vi "USRP_singlecarrierTDMUSRP1_withoutemu.vi"() -> ()   [LabVIEW 2021]
uses:
  <vilib>/addons/Modulation/Analog/controls/Complex Data Waveform.ctl
  <vilib>/Analysis/coordinate.llb/Angle Units.ctl
  <vilib>/Analysis/coordinate.llb/Angle Range (Degree).ctl
  <vilib>/Analysis/coordinate.llb/Wrap Angle (scalar).vi
  system stop.vi
  <vilib>/measure/matone.llb/Extract Single Tone Information 1 Chan (CDB).vi
  <instrlib>/niUSRP/niUSRP Fetch Rx Data (CDB Cluster).vi
  <instrlib>/niUSRP/niUSRP Write Tx Data (CDB Cluster).vi
  <vilib>/addons/Modulation/niAMT.lvlib
  <vilib>/measure/NI_MAPro.lvlib
  <vilib>/Analysis/NI_AAL_Angle.lvlib
panel:
  in  "Tab Control":T1(tab)
  in  "IQ rate Tx":dbl=400000.0 format="%#_6p"
  in  "Tx Gain":dbl format="%#_6f"
  in  "Tx IP":refnum<k15>="192.168.10.2"
  out "coerced IQ rate Tx":dbl=100000.0 format="%#_6p"
  out "coerced carrier frequency Tx":dbl=100000.0 format="%#_6p"
  in  "Rx IP":refnum<k15>="192.168.10.2"
  in  "Rx gain":dbl format="%#_6f"
  in  "Frequency":dbl=10000.0 format="%#_13g"
  in  "Duration":dbl=0.01 format="%#_13g"
  out "coerced IQ rate Rx":dbl=100000.0 format="%#_6p"
  out "coerced carrier frequency Rx":dbl=100000.0 format="%#_6p"
  in  "number of samples":i64=4000
  in  "carrier frequency":dbl=2400000000.0 format="%#_6p"
  in  "Phase in deg":dbl
  out "Waveform Graph":dbl[](graph)
  out "Boolean":bool
  out "detected frequency":dbl format="%.2p"
  out "detected Amplitude in dBm":dbl format="%.2p"
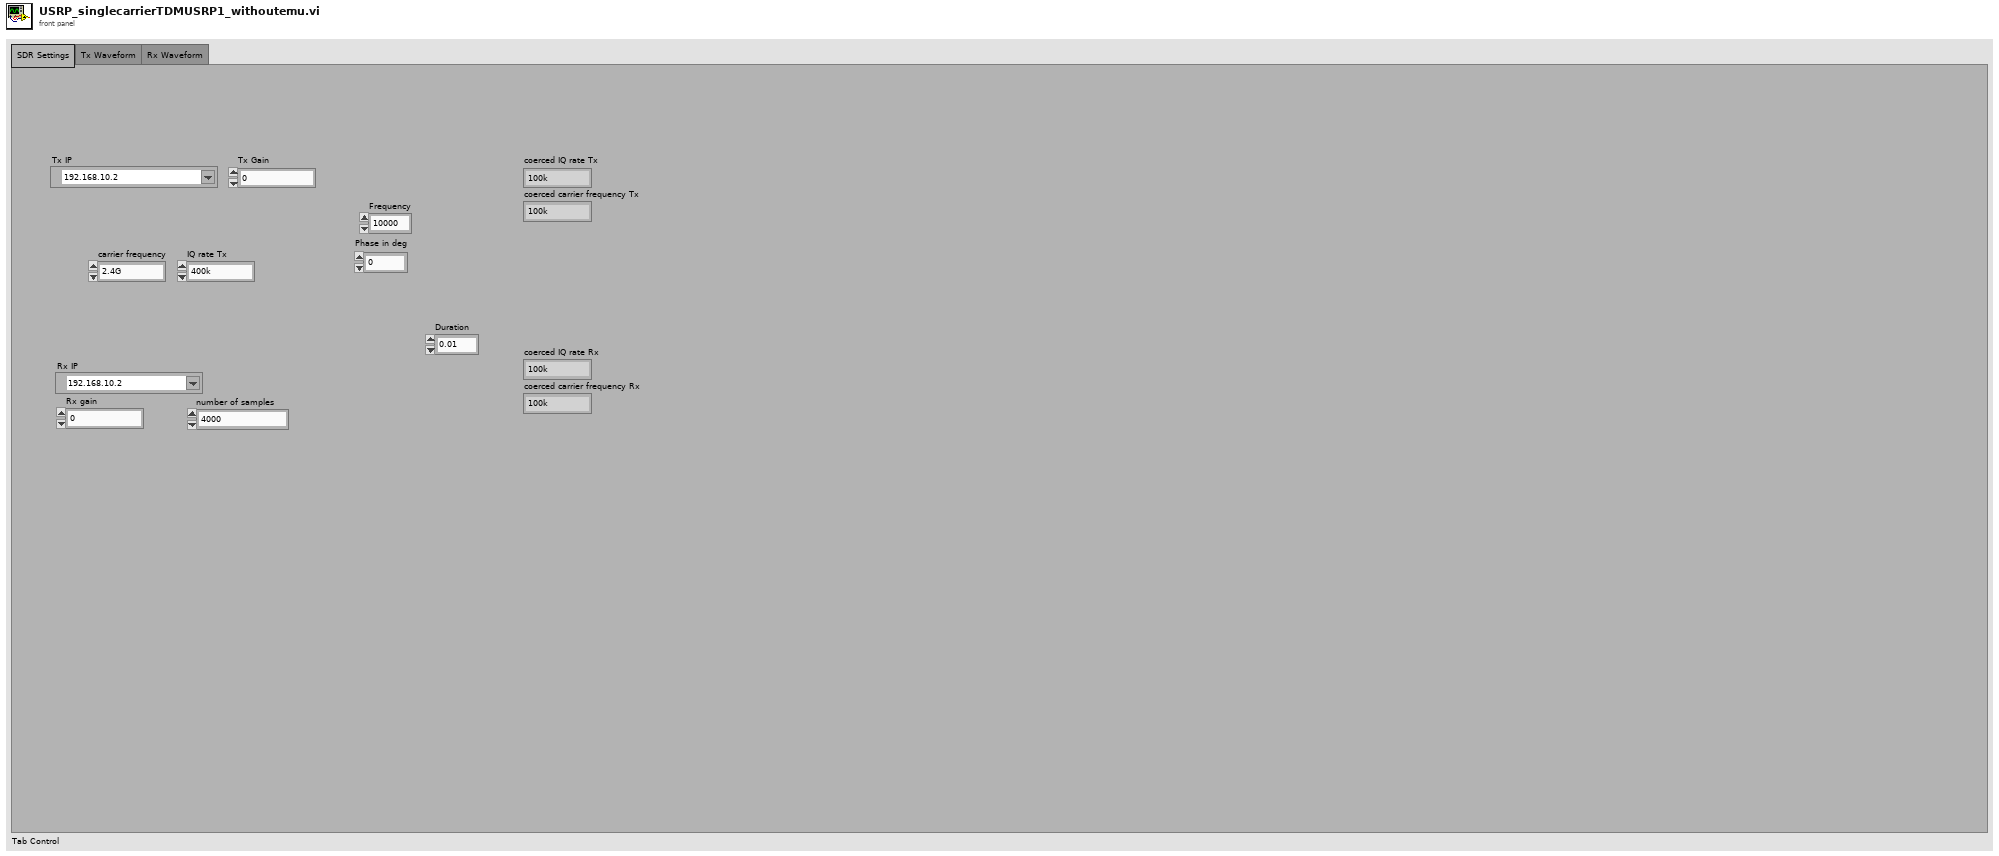
[diagram p1: front panel]
types:
  T1 = enum32{"SDR Settings", "Tx Waveform", "Rx Waveform"}
  T2 = typedef "niAMT.lvlib/Complex Data Waveform.ctl" = cluster{"t0":dbl, "dt":dbl, "Y":cdb[]}
  T3 = typedef "NI_AAL_Angle.lvlib/Angle Range (Degree).ctl" = u16
  T4 = typedef "NI_AAL_Angle.lvlib/Angle Units.ctl" = i32
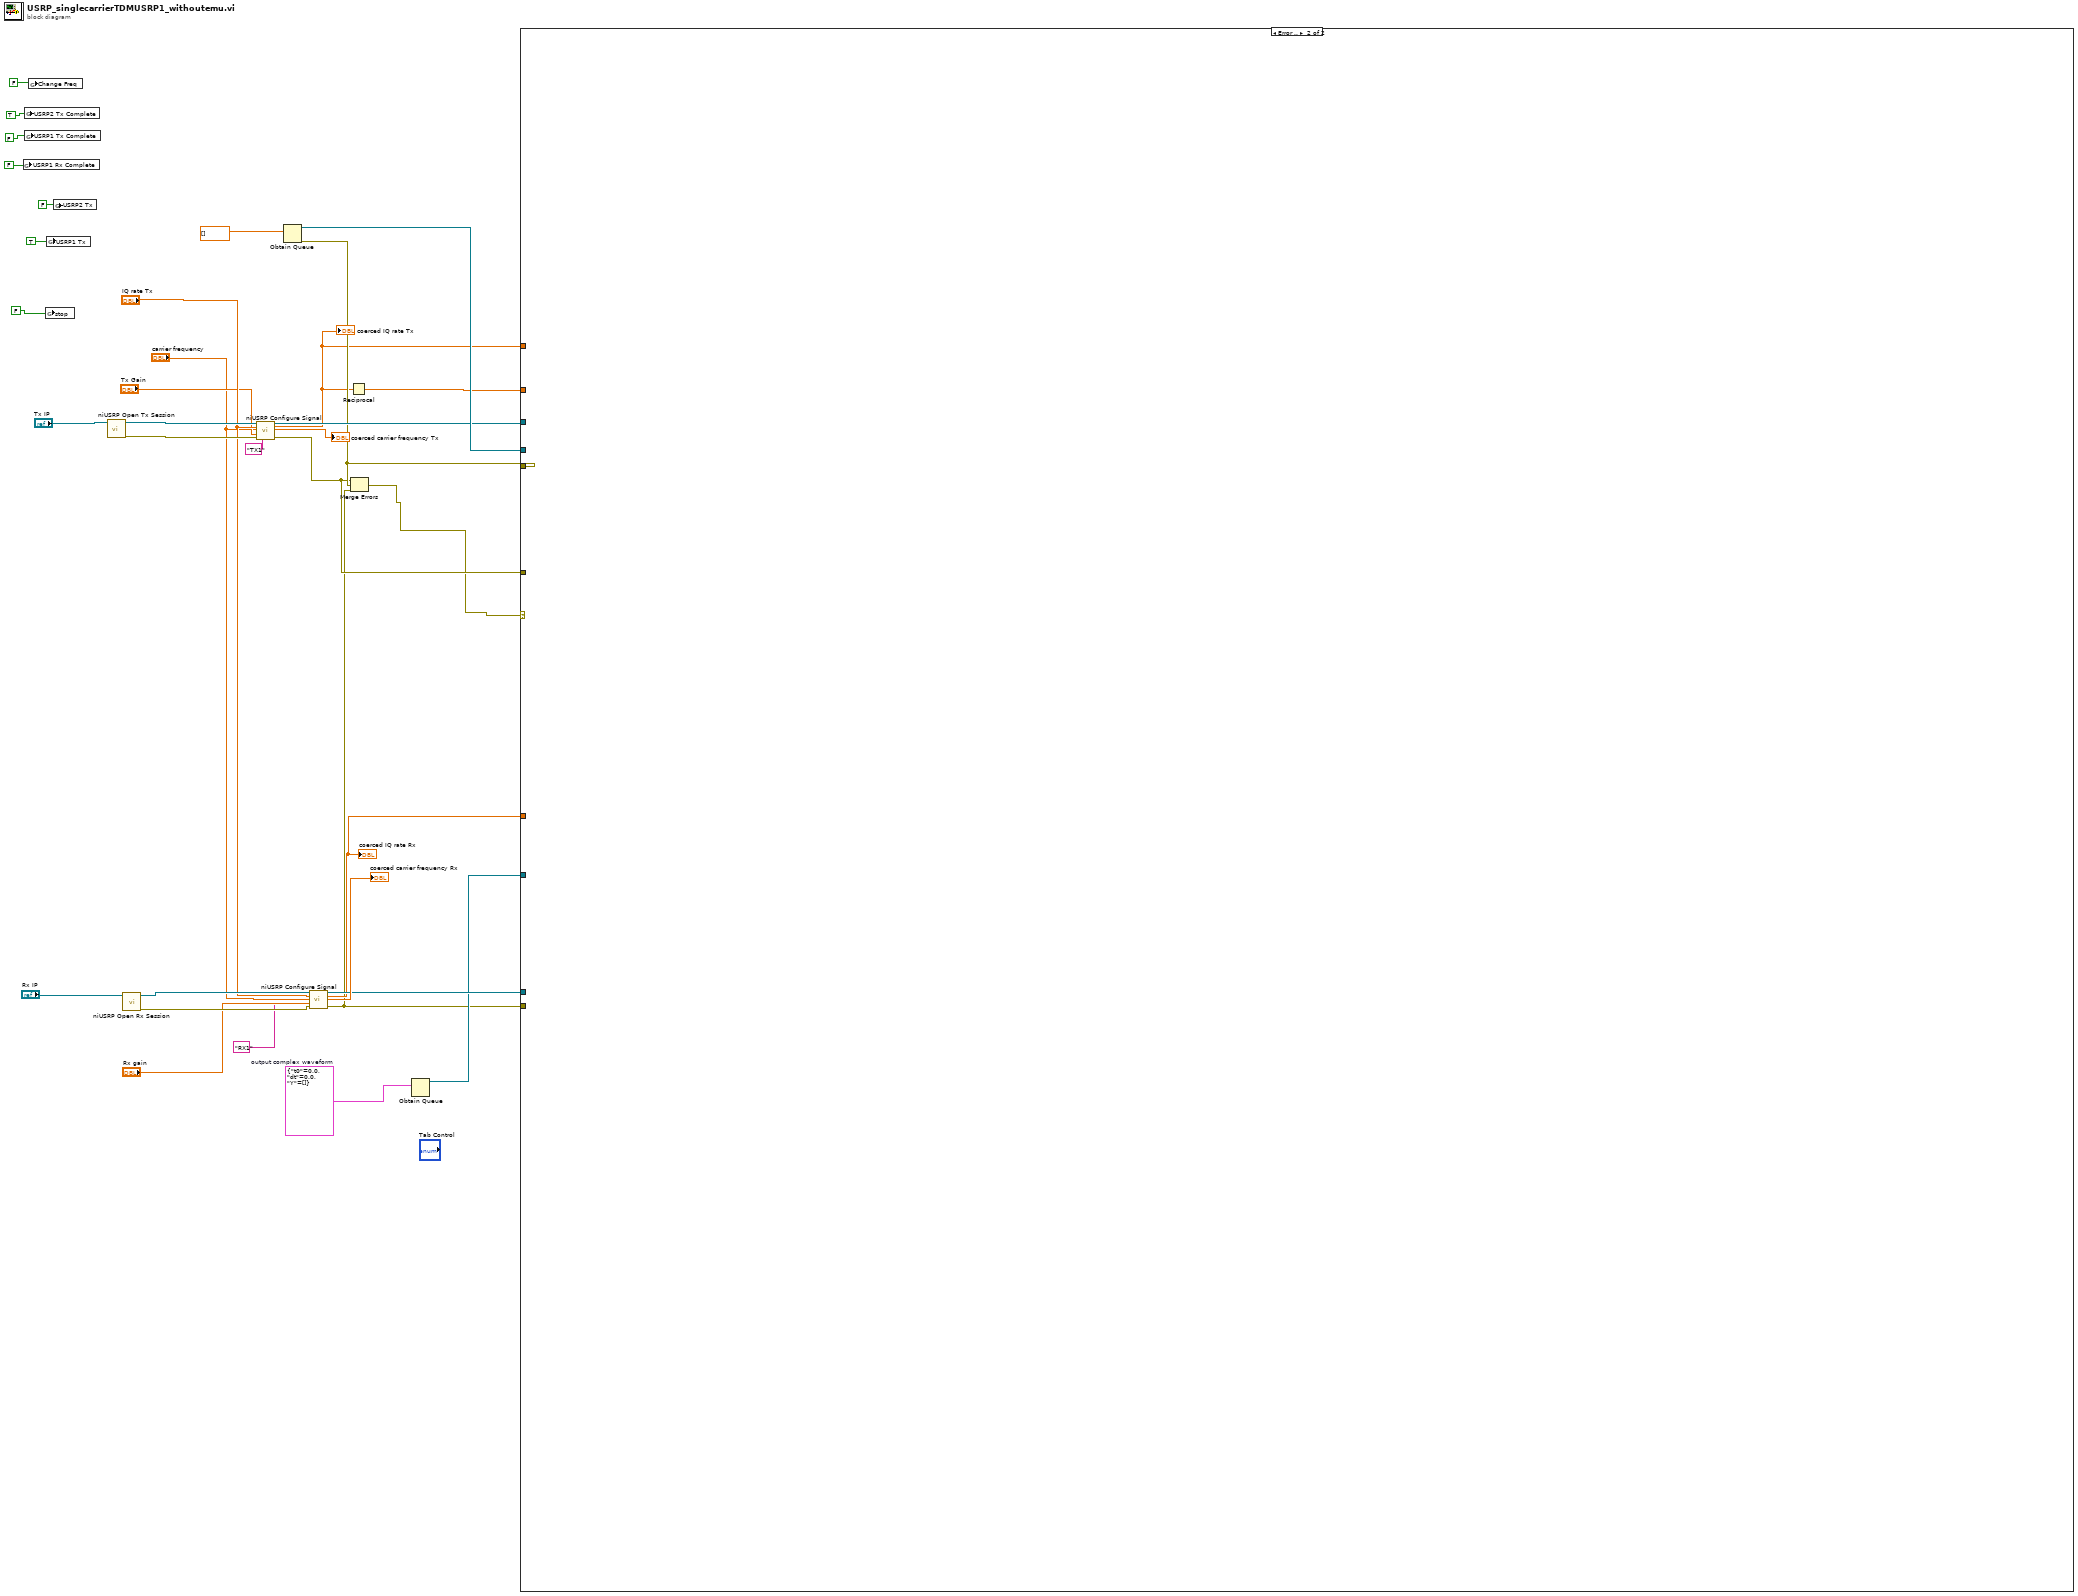
[diagram p0: block diagram]
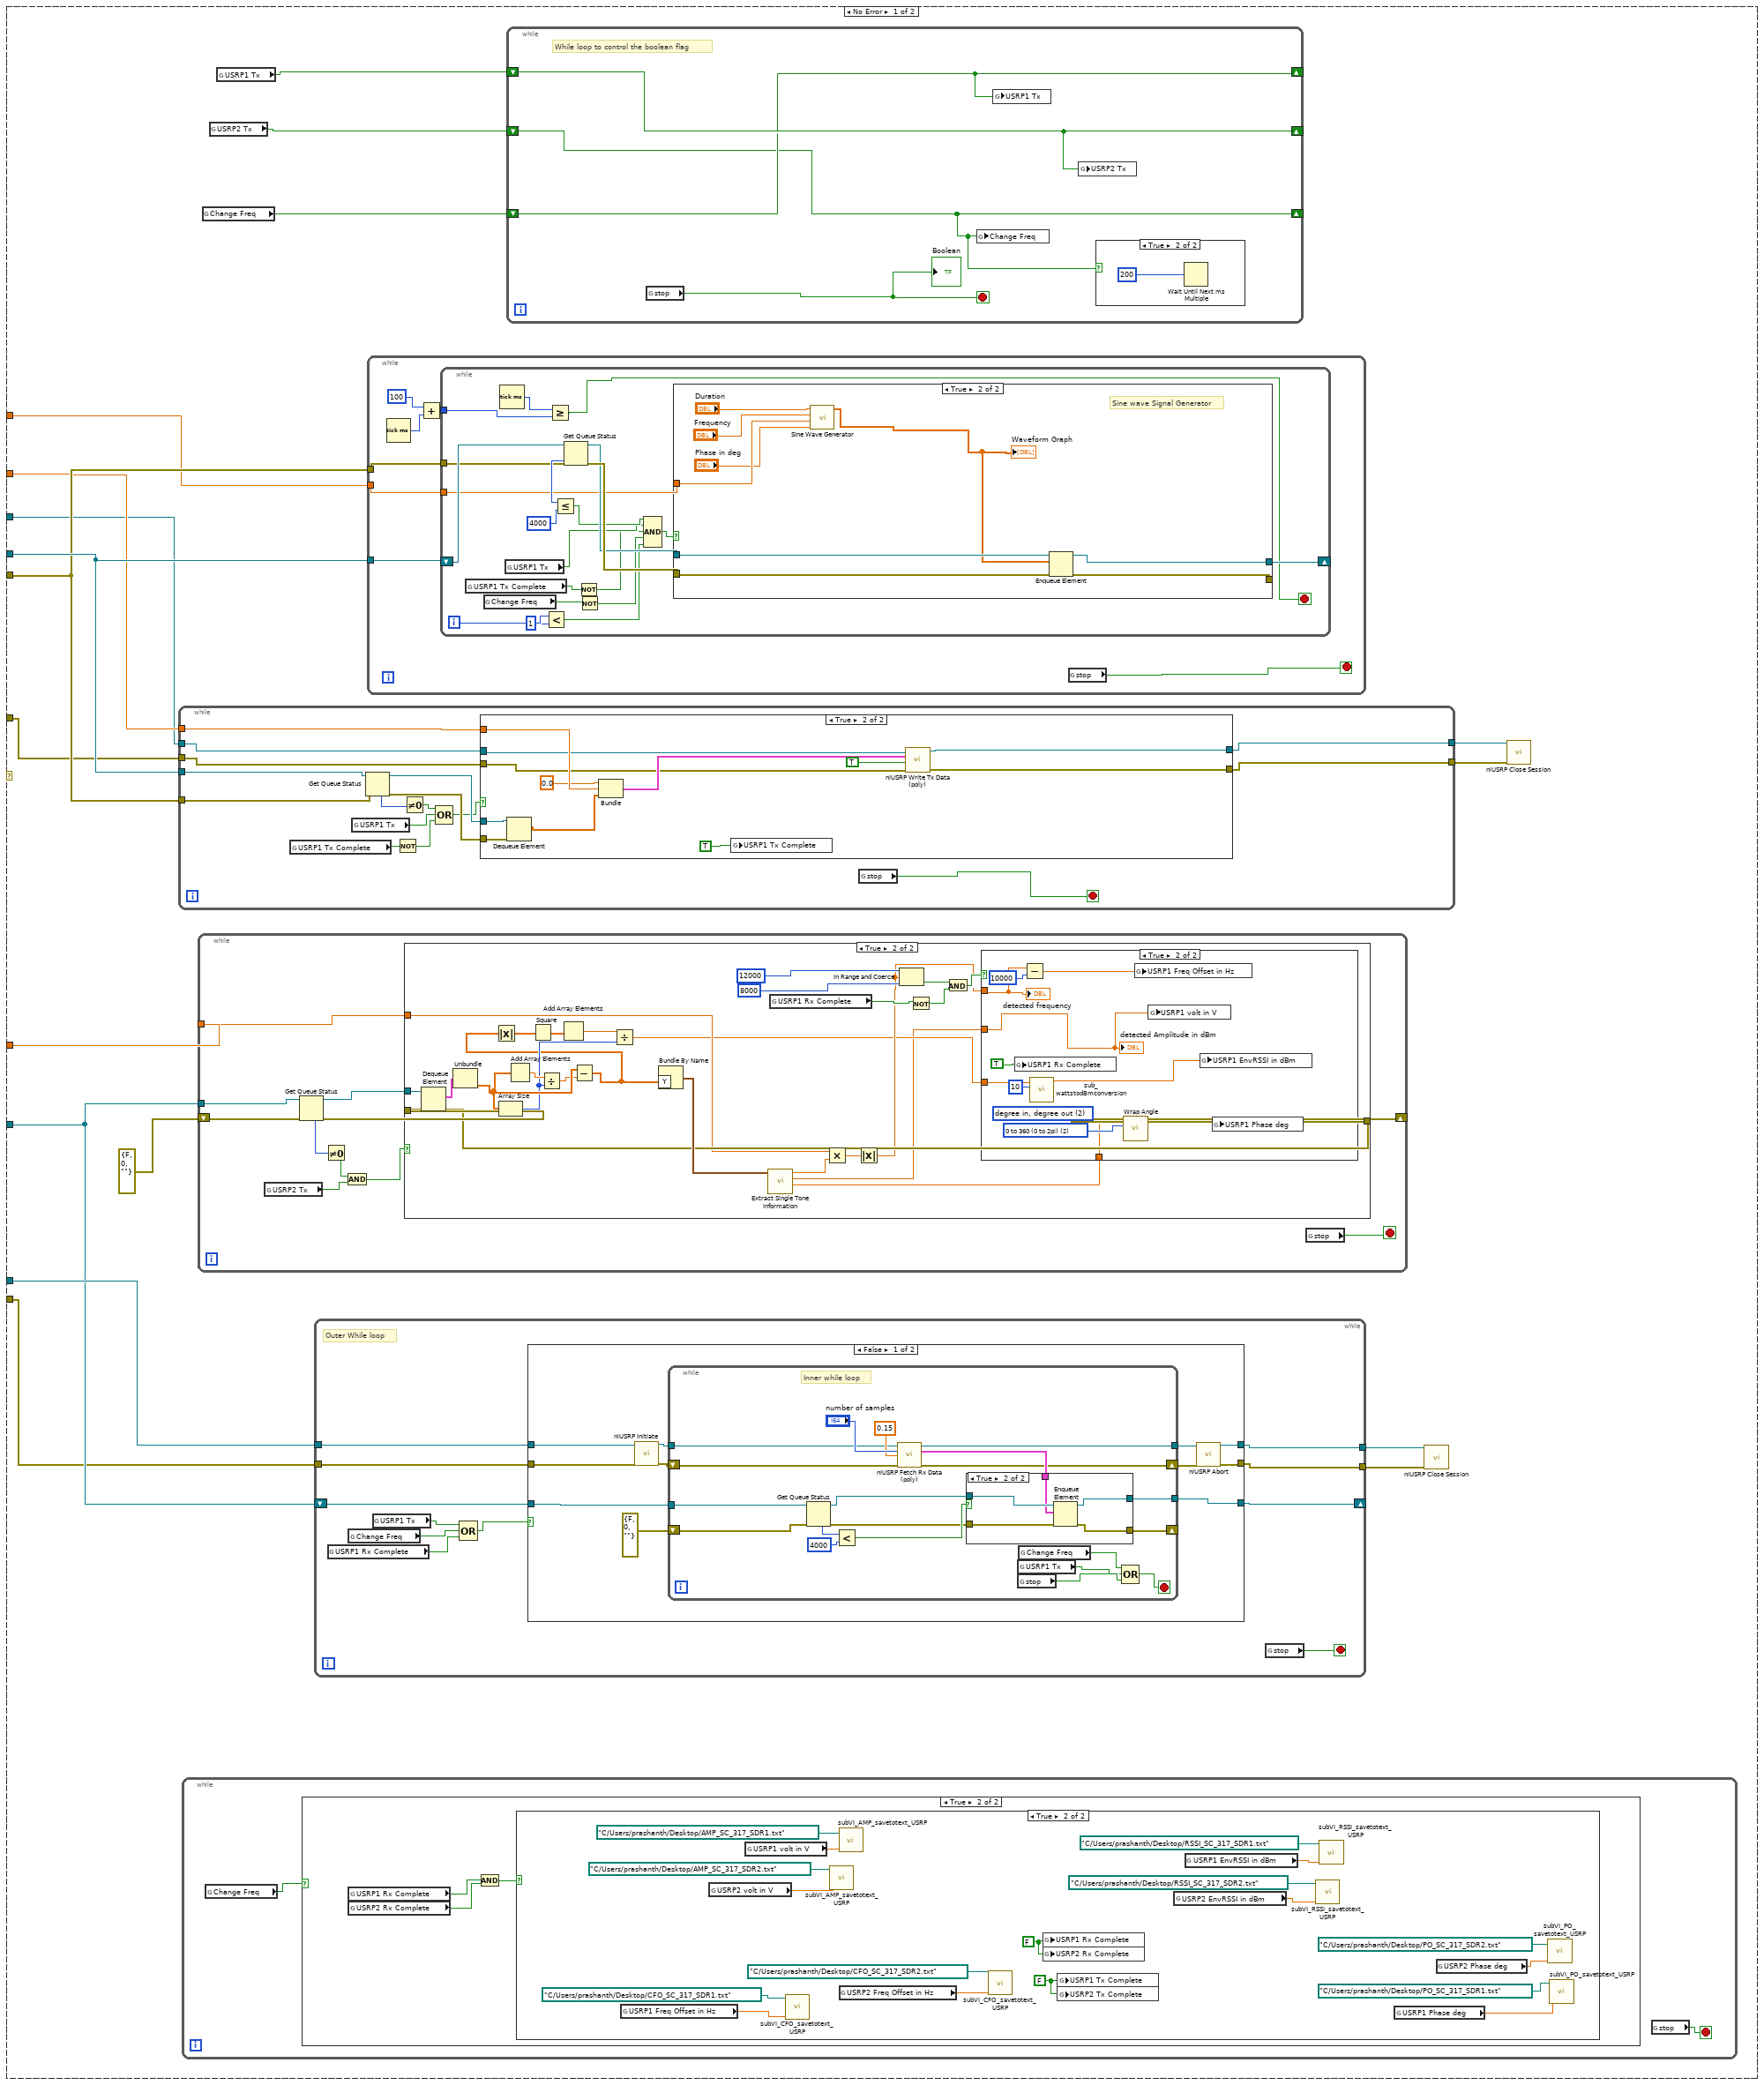
[diagram p2: hidden frame]
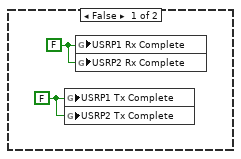
[diagram p4: hidden frame]
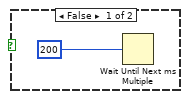
[diagram p5: hidden frame]
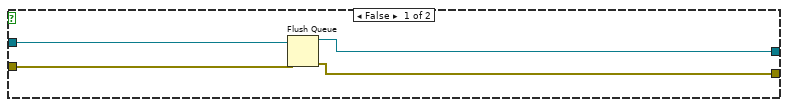
[diagram p6: hidden frame]
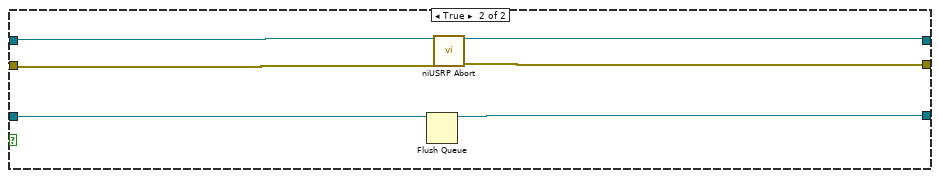
[diagram p8: hidden frame]
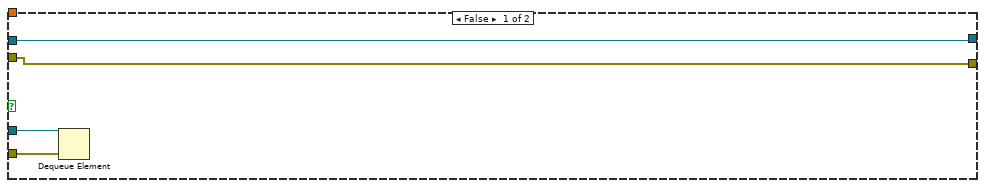
[diagram p11: hidden frame]
diagram:
  w8 = T2 {"t0"=0.0, "dt"=0.0, "Y"=[]}  # output complex waveform
  n1 = global write "system stop.vi" "USRP1 Rx Complete"(FALSE) -> ()
  n2 = global write "system stop.vi" "USRP2 Tx Complete"(TRUE) -> ()
  n3 = global write "system stop.vi" "USRP1 Tx Complete"(FALSE) -> ()
  n4 = global write "system stop.vi" "Change Freq"(FALSE) -> ()
  n5 = global write "system stop.vi" "stop"(FALSE) -> ()
  n6 = global write "system stop.vi" "USRP1 Tx"(TRUE) -> ()
  n7 = global write "system stop.vi" "USRP2 Tx"(FALSE) -> ()
  n8 = call <instrlib>:"niUSRP Open Tx Session.vi"("device names"="Tx IP") -> ("session handle out"=w33:refnum<k15>, "error out"=w32:errorcluster)  [unwired: 13 in]
  n9 = call <instrlib>:"niUSRP Open Rx Session.vi"("device names"="Rx IP") -> ("session handle out"=w30:refnum<k15>, "error out"=w29:errorcluster)  [unwired: 13 in]
  n10 = call <instrlib>:"niUSRP Configure Signal.vi"("session handle"=w33, "IQ rate"="IQ rate Tx", "carrier frequency"="carrier frequency", "gain"="Tx Gain", "error in (no error)"=w32, "active antenna"="TX1") -> ("session handle out"=w15:refnum<k15>, "coerced IQ rate"=w12:dbl, "coerced carrier frequency"=→"coerced carrier frequency Tx":dbl, "error out"=w11:errorcluster)  [unwired: 5 in, 1 out]
  "coerced IQ rate Tx" <- w12
  n11 = Obtain Queue(element data type=dbl[] []) -> (queue out=w16:refnum<queue>, error out=w13:errorcluster)  [unwired: 4 in, 1 out]
  n12 = call <instrlib>:"niUSRP Configure Signal.vi"("session handle"=w30, "IQ rate"="IQ rate Tx", "carrier frequency"="carrier frequency", "gain"="Rx gain", "error in (no error)"=w29, "active antenna"="RX1") -> ("session handle out"=w9:refnum<k15>, "coerced IQ rate"=w6:dbl, "coerced carrier frequency"=→"coerced carrier frequency Rx":dbl, "error out"=w5:errorcluster)  [unwired: 5 in, 1 out]
  "coerced IQ rate Rx" <- w6
  n13 = Reciprocal(x=w12) -> (1/x=w14:dbl)
  n14 = Merge Errors(w11, w13, w5) -> (w3:errorcluster)
  n15 = Obtain Queue(element data type=w8) -> (queue out=w7:refnum<queue>)  [unwired: 4 in, 2 out]
  n16 = case shown="Error .." w3 {
    tunnel: w13 -> [w51 _]
    tunnel: w16 -> [w52 _]
    tunnel: w15 -> [w49 _]
    tunnel: w14 -> [w50 _]
    tunnel: w12 -> [w48 _]
    tunnel: w11 -> [w47 _]
    tunnel: w9 -> [w45 _]
    tunnel: w7 -> [w44 _]
    tunnel: w6 -> [w43 _]
    tunnel: w5 -> [w42 _]
    frame No Error {
      n17 = while {
        tunnel: w52 -> [w245]
        tunnel: w51 -> [w242]
        tunnel: w50 -> [w241]
        tunnel: w49 -> [w238]
        tunnel: w47 -> [w237]
        tunnel: [w231] -> w38
        tunnel: [w230] -> w37
        stop <- w239 stop-if-true
        n18 = global read "system stop.vi" "USRP1 Tx Complete"() -> (w233:bool)
        n19 = global read "system stop.vi" "USRP1 Tx"() -> (w235:bool)
        n20 = Get Queue Status(queue=w245, error in (no error)=w242) -> (queue out=w244:refnum<queue>, error out=w243:errorcluster, # elements in queue=w240:i32)  [unwired: 1 in, 5 out]
        n21 = Not(x=w233) -> (.not. x?=w234:bool)
        n22 = Not Equal To 0?(x=w240) -> (x != 0?=w236:bool)
        n23 = Compound Arithmetic op=OR(w236, w235, w234) -> (w232:bool)
        n24 = case shown="True" w232 {
          tunnel: w244 -> [w247 w261]
          tunnel: w243 -> [w246 w260]
          tunnel: w241 -> [_ w259]
          tunnel: w238 -> [w249 w252]
          tunnel: w237 -> [w248 w251]
          tunnel: [w249 w255] -> w231
          tunnel: [w248 w253] -> w230
          frame False {
            n25 = Dequeue Element(queue=w247, error in (no error)=w246) -> ()  [unwired: 1 in, 4 out]
          }
          frame True {
            n26 = Dequeue Element(queue=w261, error in (no error)=w260) -> (element=w250:dbl[])  [unwired: 1 in, 3 out]
            n27 = Bundle(0.0, w259, w250) -> (w258:cluster{dbl, dbl, dbl[]})  [unwired: 1 in]
            n28 = global write "system stop.vi" "USRP1 Tx Complete"(TRUE) -> ()
            n29 = call-poly <instrlib>:"niUSRP Write Tx Data (poly).vi"("session handle"=w252, "data"=w258, "end of data?"=TRUE, "error in (no error)"=w251) -> ("session handle out"=w255:refnum<k15>, "error out"=w253:errorcluster)  [unwired: 10 in]
          }
        }
        n30 = global read "system stop.vi" "stop"() -> (w239:bool)
      }
      n31 = while {
        stop <- w53 stop-if-true
        n32 = global read "system stop.vi" "Change Freq"() -> (w54:bool)
        n33 = case shown="True" w54 {
          frame False {
          }
          frame True {
            n34 = global read "system stop.vi" "USRP1 Rx Complete"() -> (w57:bool)
            n35 = global read "system stop.vi" "USRP2 Rx Complete"() -> (w56:bool)
            n36 = And(x=w57, y=w56) -> (x .and. y?=w55:bool)
            n37 = case shown="True" w55 {
              frame False {
                w59 = FALSE
                w58 = FALSE
                n38 = global write "system stop.vi" "USRP1 Tx Complete"(w59) -> ()
                n39 = global write "system stop.vi" "USRP2 Tx Complete"(w59) -> ()
                n40 = global write "system stop.vi" "USRP1 Rx Complete"(w58) -> ()
                n41 = global write "system stop.vi" "USRP2 Rx Complete"(w58) -> ()
              }
              frame True {
                w77 = FALSE
                w76 = FALSE
                n42 = global read "system stop.vi" "USRP1 Freq Offset in Hz"() -> (w70:dbl)
                n43 = global read "system stop.vi" "USRP2 volt in V"() -> (w73:dbl)
                n44 = global read "system stop.vi" "USRP1 volt in V"() -> (w74:dbl)
                n45 = call "subVI_CFO_savetotext_USRP.vi"("RSSI"=w70, "file path (dialog if empty)"=path "C:/Users/prashanth/Desktop/CFO_SC_317_SDR1.txt") -> ()  [unwired: 10 in]
                n46 = call "subVI_AMP_savetotext_USRP.vi"("RSSI"=w73, "file path (dialog if empty)"=path "C:/Users/prashanth/Desktop/AMP_SC_317_SDR2.txt") -> ()  [unwired: 10 in]
                n47 = call "subVI_AMP_savetotext_USRP.vi"("RSSI"=w74, "file path (dialog if empty)"=path "C:/Users/prashanth/Desktop/AMP_SC_317_SDR1.txt") -> ()  [unwired: 10 in]
                n48 = global read "system stop.vi" "USRP2 Freq Offset in Hz"() -> (w68:dbl)
                n49 = call "subVI_CFO_savetotext_USRP.vi"("RSSI"=w68, "file path (dialog if empty)"=path "C:/Users/prashanth/Desktop/CFO_SC_317_SDR2.txt") -> ()  [unwired: 10 in]
                n50 = global write "system stop.vi" "USRP1 Rx Complete"(w76) -> ()
                n51 = global write "system stop.vi" "USRP2 Rx Complete"(w76) -> ()
                n52 = global write "system stop.vi" "USRP1 Tx Complete"(w77) -> ()
                n53 = global write "system stop.vi" "USRP2 Tx Complete"(w77) -> ()
                n54 = global read "system stop.vi" "USRP2 EnvRSSI in dBm"() -> (w66:dbl)
                n55 = global read "system stop.vi" "USRP1 EnvRSSI in dBm"() -> (w64:dbl)
                n56 = call "subVI_RSSI_savetotext_USRP.vi"("RSSI"=w66, "file path (dialog if empty)"=path "C:/Users/prashanth/Desktop/RSSI_SC_317_SDR2.txt") -> ()  [unwired: 10 in]
                n57 = call "subVI_RSSI_savetotext_USRP.vi"("RSSI"=w64, "file path (dialog if empty)"=path "C:/Users/prashanth/Desktop/RSSI_SC_317_SDR1.txt") -> ()  [unwired: 10 in]
                n58 = global read "system stop.vi" "USRP1 Phase deg"() -> (w62:dbl)
                n59 = global read "system stop.vi" "USRP2 Phase deg"() -> (w60:dbl)
                n60 = call "subVI_PO_savetotext_USRP.vi"("RSSI"=w60, "file path (dialog if empty)"=path "C:/Users/prashanth/Desktop/PO_SC_317_SDR2.txt") -> ()  [unwired: 10 in]
                n61 = call "subVI_PO_savetotext_USRP.vi"("RSSI"=w62, "file path (dialog if empty)"=path "C:/Users/prashanth/Desktop/PO_SC_317_SDR1.txt") -> ()  [unwired: 10 in]
              }
            }
          }
        }
        n62 = global read "system stop.vi" "stop"() -> (w53:bool)
      }
      n63 = while {
        tunnel: w44 -> [w187]
        shift-right: [w185] -> _
        shift-left: errorcluster {"status"=FALSE, "code"=0, "source"=""} ("error in (no error)") -> [w186]
        tunnel: w43 -> [w184]
        stop <- w183 stop-if-true
        n64 = global read "system stop.vi" "USRP2 Tx"() -> (w182:bool)
        n65 = Get Queue Status(queue=w187, error in (no error)=w186) -> (queue out=w189:refnum<queue>, error out=w188:errorcluster, # elements in queue=w190:i32)  [unwired: 1 in, 5 out]
        n66 = Not Equal To 0?(x=w190) -> (x != 0?=w181:bool)
        n67 = And(x=w181, y=w182) -> (x .and. y?=w180:bool)
        n68 = case shown="True" w180 {
          tunnel: w189 -> [_ w217]
          tunnel: w188 -> [w191 w216]
          tunnel: [w191 w206] -> w185
          tunnel: w184 -> [_ w204]
          frame False {
          }
          frame True {
            n69 = Dequeue Element(queue=w217, error in (no error)=w216) -> (element=w215:T2, error out=w206:errorcluster)  [unwired: 1 in, 2 out]
            n70 = Unbundle(w215) -> ("Y"=w201:cdb[])  [unwired: 2 out]
            n71 = Array Size(array=w201) -> (size(s)=w198:i32)
            n72 = Add Array Elements(numeric array=w201) -> (sum=w214:cdb)
            n73 = Divide(x=w214, y=w198) -> (x/y=w199:cdb)
            n74 = Subtract(x=w201, y=w199) -> (x-y=w193:cdb[])
            n75 = Absolute Value(x=w193) -> (abs(x)=w200:dbl[])
            n76 = Square(x=w200) -> (x^2=w197:dbl[])
            n77 = Add Array Elements(numeric array=w197) -> (sum=w196:dbl)
            n78 = Divide(x=w196, y=w198) -> (x/y=w195:dbl)
            n79 = Bundle By Name("Y"=w193) -> (w207:waveform(cdb))  [unwired: 1 in]
            n80 = call-poly <vilib>:"Extract Single Tone Information.vi"("time signal in"=w207) -> ("detected phase (deg)"=w194:dbl, "detected amplitude"=w192:dbl, "detected frequency"=w205:dbl)  [unwired: 5 in, 3 out]
            n81 = global read "system stop.vi" "USRP1 Rx Complete"() -> (w209:bool)
            n82 = Multiply(x=w204, y=w205) -> (x*y=w203:dbl)
            n83 = Absolute Value(x=w203) -> (abs(x)=w202:dbl)
            n84 = In Range and Coerce(upper limit=12000, x=w202, lower limit=8000) -> (In Range?=w210:bool)  [unwired: 1 out]
            n85 = Not(x=w209) -> (.not. x?=w208:bool)
            n86 = And(x=w210, y=w208) -> (x .and. y?=w211:bool)
            n87 = case shown="True" w211 {
              tunnel: w202 -> [_ w228]
              tunnel: w192 -> [_ w218]
              tunnel: w195 -> [_ w225]
              tunnel: w194 -> [_ w220]
              frame False {
              }
              frame True {
                w222 = T3 2 items=["none", "-180 to 180 (-pi to pi)", "0 to 360 (0 to 2pi)"] ("angle range")
                w223 = T4 2 items=["radian in, radian out", "radian in, degree out", "degree in, degree out", "degree in, radian out"] ("angle units")
                n88 = global write "system stop.vi" "USRP1 Rx Complete"(TRUE) -> ()
                n89 = Subtract(x=w228, y=10000) -> (x-y=w226:dbl)
                n90 = call "sub_wattstodBmconversion.vi"("Amp or Power"=10, "detected amplitude"=w225) -> ("Numeric"=w224:dbl)  [unwired: 9 in]
                n91 = call-poly <vilib>:"Wrap Angle.vi"("angle units"=w223, "angle range"=w222, "angle in"=w220) -> ("angle out"=w221:dbl)  [unwired: 7 in, 1 out]
                n92 = global write "system stop.vi" "USRP1 Freq Offset in Hz"(w226) -> ()
                n93 = global write "system stop.vi" "USRP1 volt in V"(w218) -> ()
                n94 = global write "system stop.vi" "USRP1 EnvRSSI in dBm"(w224) -> ()
                n95 = global write "system stop.vi" "USRP1 Phase deg"(w221) -> ()
                "detected frequency" <- w228
                "detected Amplitude in dBm" <- w218
              }
            }
          }
        }
        n96 = global read "system stop.vi" "stop"() -> (w183:bool)
      }
      n97 = global read "system stop.vi" "Change Freq"() -> (w40:bool)
      n98 = global read "system stop.vi" "USRP2 Tx"() -> (w39:bool)
      n99 = global read "system stop.vi" "USRP1 Tx"() -> (w41:bool)
      n100 = while {
        shift-right: [w131] -> _
        shift-left: w44 -> [w135]
        tunnel: w45 -> [w133]
        tunnel: w42 -> [w132]
        tunnel: [w126] -> w36
        tunnel: [w125] -> w35
        stop <- w134 stop-if-true
        # "Outer While loop"
        n101 = global read "system stop.vi" "USRP1 Rx Complete"() -> (w129:bool)
        n102 = global read "system stop.vi" "Change Freq"() -> (w127:bool)
        n103 = global read "system stop.vi" "USRP1 Tx"() -> (w128:bool)
        n104 = Compound Arithmetic op=OR(w128, w127, w129) -> (w130:bool)
        n105 = case shown="False" w130 {
          tunnel: w133 -> [w138 w179]
          tunnel: w135 -> [w146 w175]
          tunnel: w132 -> [w137 w177]
          tunnel: [w141 w178] -> w126
          tunnel: [w140 w176] -> w125
          tunnel: [w136 w174] -> w131
          frame False {
            n106 = call <instrlib>:"niUSRP Initiate.vi"("session handle"=w138, "error in (no error)"=w137) -> ("session handle out"=w144:refnum<k15>, "error out"=w143:errorcluster)  [unwired: 12 in]
            n107 = while {
              tunnel: w146 -> [w166]
              shift-right: [w150] -> w139
              shift-left: w143 -> [w152]
              shift-right: [w165] -> _
              shift-left: errorcluster {"status"=FALSE, "code"=0, "source"=""} ("error in (no error)") -> [w164]
              tunnel: w144 -> [w153]
              tunnel: [w151] -> w142
              tunnel: [w147] -> w136
              stop <- w156 stop-if-true
              # "Inner while loop"
              n108 = Get Queue Status(queue=w166, error in (no error)=w164) -> (queue out=w159:refnum<queue>, error out=w160:errorcluster, # elements in queue=w163:i32)  [unwired: 1 in, 5 out]
              n109 = Less?(x=w163, y=4000) -> (x < y?=w161:bool)
              n110 = call-poly <instrlib>:"niUSRP Fetch Rx Data (poly).vi"("session handle"=w153, "number of samples"="number of samples", "timeout"=0.15, "error in (no error)"=w152) -> ("session handle out"=w151:refnum<k15>, "data"=w157:cluster{"t0":dbl, "dt":dbl, "Y":cdb[]}, "error out"=w150:errorcluster)  [unwired: 8 in, 1 out]
              n111 = case shown="True" w161 {
                tunnel: w160 -> [w168 w173]
                tunnel: w159 -> [w167 w172]
                tunnel: w157 -> [_ w171]
                tunnel: [w168 w170] -> w165
                tunnel: [w167 w169] -> w147
                frame False {
                }
                frame True {
                  n112 = Enqueue Element(queue=w172, element=w171, error in (no error)=w173) -> (queue out=w169:refnum<queue>, error out=w170:errorcluster)  [unwired: 1 in, 1 out]
                }
              }
              n113 = global read "system stop.vi" "USRP1 Tx"() -> (w149:bool)
              n114 = global read "system stop.vi" "stop"() -> (w155:bool)
              n115 = global read "system stop.vi" "Change Freq"() -> (w148:bool)
              n116 = Compound Arithmetic op=OR(w148, w149, w155) -> (w156:bool)
            }
            n117 = call <instrlib>:"niUSRP Abort.vi"("session handle"=w142, "error in (no error)"=w139) -> ("session handle out"=w141:refnum<k15>, "error out"=w140:errorcluster)  [unwired: 12 in]
          }
          frame True {
            n118 = Flush Queue(queue=w175) -> (queue out=w174:refnum<queue>)  [unwired: 1 in, 2 out]
            n119 = call <instrlib>:"niUSRP Abort.vi"("session handle"=w179, "error in (no error)"=w177) -> ("session handle out"=w178:refnum<k15>, "error out"=w176:errorcluster)  [unwired: 12 in]
          }
        }
        n120 = global read "system stop.vi" "stop"() -> (w134:bool)
      }
      n121 = while {
        tunnel: w51 -> [w89]
        tunnel: w48 -> [w88]
        tunnel: w52 -> [w90]
        stop <- w84 stop-if-true
        n122 = Tick Count (ms)() -> (millisecond timer value=w86:u32)
        n123 = Add(x=100, y=w86) -> (x+y=w85:u32)
        n124 = while {
          tunnel: w89 -> [w106]
          tunnel: w88 -> [w105]
          tunnel: w85 -> [w100]
          shift-right: [w98] -> _
          shift-left: w90 -> [w107]
          i -> [w93]
          stop <- w95 stop-if-true
          n125 = global read "system stop.vi" "USRP1 Tx Complete"() -> (w97:bool)
          n126 = global read "system stop.vi" "Change Freq"() -> (w96:bool)
          n127 = Tick Count (ms)() -> (millisecond timer value=w101:u32)
          n128 = global read "system stop.vi" "USRP1 Tx"() -> (w103:bool)
          n129 = Less?(x=w93, y=1) -> (x < y?=w91:bool)
          n130 = Greater Or Equal?(x=w101, y=w100) -> (x >= y?=w95:bool)
          n131 = Get Queue Status(queue=w107, error in (no error)=w106) -> (queue out=w108:refnum<queue>, error out=w109:errorcluster, # elements in queue=w111:i32)  [unwired: 1 in, 5 out]
          n132 = Less Or Equal?(x=w111, y=4000) -> (x <= y?=w104:bool)
          n133 = Not(x=w97) -> (.not. x?=w99:bool)
          n134 = Not(x=w96) -> (.not. x?=w94:bool)
          n135 = Compound Arithmetic op=AND(w104, w103, w99, w94, w91) -> (w102:bool)
          n136 = case shown="True" w102 {
            tunnel: w109 -> [w114 w124]
            tunnel: w108 -> [w115 w123]
            tunnel: w105 -> [_ w119]
            tunnel: [w113 w121] -> w98
            tunnel: [w112 w116] -> _
            frame False {
              n137 = Flush Queue(queue=w115, error in (no error)=w114) -> (queue out=w113:refnum<queue>, error out=w112:errorcluster)  [unwired: 1 out]
            }
            frame True {
              # "Sine wave Signal Generator"
              n138 = call "SIne Wave Generator.vi"("Phase in deg"="Phase in deg", "Sampling rate"=w119, "Frequency"="Frequency", "Duration"="Duration") -> ("Array"=w117:dbl[])  [unwired: 6 in, 1 out]
              "Waveform Graph" <- w117
              n139 = Enqueue Element(queue=w123, element=w117, error in (no error)=w124) -> (queue out=w121:refnum<queue>, error out=w116:errorcluster)  [unwired: 1 in, 1 out]
            }
          }
        }
        n140 = global read "system stop.vi" "stop"() -> (w84:bool)
      }
      n141 = while {
        shift-right: [w79] -> _
        shift-left: w41 -> [w81]
        shift-right: [w81] -> _
        shift-left: w39 -> [w78]
        shift-right: [w78] -> _
        shift-left: w40 -> [w79]
        stop <- w80 stop-if-true
        # "While loop to control the boolean flag"
        n142 = global read "system stop.vi" "stop"() -> (w80:bool)
        "Boolean" <- w80
        n143 = global write "system stop.vi" "Change Freq"(w78) -> ()
        n144 = global write "system stop.vi" "USRP1 Tx"(w79) -> ()
        n145 = global write "system stop.vi" "USRP2 Tx"(w81) -> ()
        n146 = case shown="True" w78 {
          frame False {
            n147 = Wait Until Next ms Multiple(millisecond multiple=200) -> ()  [unwired: 1 out]
          }
          frame True {
            n148 = Wait Until Next ms Multiple(millisecond multiple=200) -> ()  [unwired: 1 out]
          }
        }
      }
      n149 = call <instrlib>:"niUSRP Close Session.vi"("session handle"=w36, "error in (no error)"=w35) -> ()  [unwired: 13 in, 1 out]
      n150 = call <instrlib>:"niUSRP Close Session.vi"("session handle"=w38, "error in (no error)"=w37) -> ()  [unwired: 13 in, 1 out]
    }
    frame Error {
    }
  }
